vi "Main - Add EtherCAT Master.vi"(8 "error in (no error)":errorcluster, 11 "Node Ptr":u64 format="%.0x") -> (0 "error out":errorcluster)   [LabVIEW 2019, in "SEECD System Explorer.lvlib"]
uses:
  SEECD System Explorer.lvlib
  Shared/Globals/Scan Engine GUIDs.vi
  Shared/Globals/Property Strings.vi
  <vilib>/NI VeriStand/Custom Device API/Custom Device API.lvlib
  Shared/SEECD Shared.lvlib
panel:
  in  "Tag":string
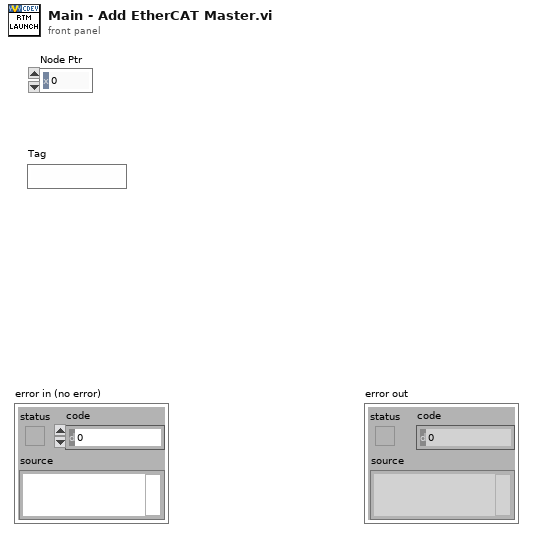
[diagram p1: front panel]
types:
  T1 = typedef "Custom Device API.lvlib/Custom Device Item Ref.ctl" = u64
  T2 = typedef "Custom Device API.lvlib/Custom Device Item Info.ctl" = cluster{"Name":string, "Is Channel":bool, "GUID":string, "Is Waveform":bool}
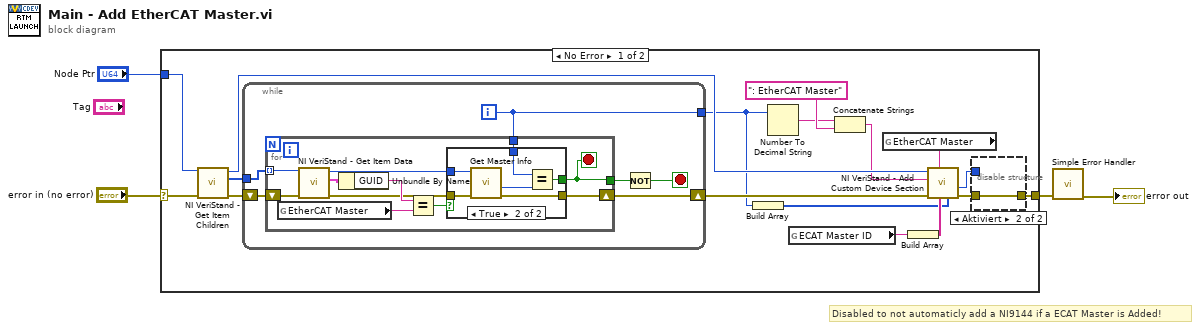
[diagram p0: block diagram]
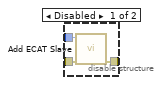
[diagram p2: hidden frame]
diagram:
  # "Disabled to not automaticly add a NI9144 if a ECAT Master is Added!"
  n1 = case shown="No Error" "error in (no error)" {
    selector: "error in (no error)" -> [w21 w50]
    tunnel: "Node Ptr" -> [w20 _]
    tunnel: [w19 w50] -> w2
    frame No Error {
      n2 = call <vilib>:"NI VeriStand - Get Item Children.vi"("error in (no error)"=w21, "Item Ref in"=w20) -> ("error out"=w18:errorcluster, "Child Refs"=w17:T1[], "Item Ref out"=w14:T1)  [unwired: 6 in, 1 out]
      n3 = while {
        shift-right: [w27] -> w15
        shift-left: w18 -> [w31]
        tunnel: w17 -> [w30]
        tunnel: [w26] -> w10
        i -> [w26]
        stop <- w28 stop-if-true
        n4 = for {
          tunnel: w30 -> [w37] mode=indexing
          shift-right: [w40] -> w27
          shift-left: w31 -> [w38]
          tunnel: w26 -> [w42]
          tunnel: [w41] -> w29
          stop <- w41 stop-if-true
          n5 = global read "Scan Engine GUIDs.vi" "EtherCAT Master"() -> (w35:string)
          n6 = call <vilib>:"NI VeriStand - Get Item Data.vi"("error in (no error)"=w38, "Item Ref in"=w37) -> ("error out"=w34:errorcluster, "Item Info"=w39:T2, "Item Ref out"=w33:T1)  [unwired: 6 in, 1 out]
          n7 = Unbundle By Name(w39) -> ("GUID"=w36:string)
          n8 = Equal?(x=w36, y=w35) -> (x = y?=w32:bool)
          n9 = case shown="True" w32 {
            tunnel: w42 -> [_ w49]
            tunnel: [_ w48] -> w41
            tunnel: [w43 w47] -> w40
            tunnel: w34 -> [w43 w45]
            tunnel: w33 -> [_ w44]
            frame False {
            }
            frame True {
              n10 = call "Get Master Info.vi"("error in (no error)"=w45, "Item Ref in"=w44) -> ("error out"=w47:errorcluster, "Master #"=w46:u32)  [unwired: 6 in, 2 out]
              n11 = Equal?(x=w49, y=w46) -> (x = y?=w48:bool)
            }
          }
        }
        n12 = Not(x=w29) -> (.not. x?=w28:bool)
      }
      n13 = Build Array(w10) -> (w11:i32[])
      n14 = Number To Decimal String(number=w10) -> (decimal integer string=w8:string)  [unwired: 1 in]
      n15 = global read "Property Strings.vi" "ECAT Master ID"() -> (w13:string)
      n16 = Concatenate Strings(w8, ": EtherCAT Master" ("string")) -> (w7:string)
      n17 = global read "Scan Engine GUIDs.vi" "EtherCAT Master"() -> (w16:string)
      n18 = Build Array(w13) -> (w12:string[])
      n19 = call <vilib>:"NI VeriStand - Add Custom Device Section.vi"("Property Values"=w11, "Property names"=w12, "GUID (Default Section)"=w16, "error in (no error)"=w15, "Section Name"=w7, "Parent Ref in"=w14) -> ("error out"=w6:errorcluster, "Section Ptr"=w5:T1)  [unwired: 2 in, 2 out]
      n20 = disable-structure shown="Aktiviert" {
        disable-tunnel: [w24 w25] -> w19
        disable-tunnel: w6 -> [w23 w25]
        disable-tunnel: w5 -> [w22 _]
        frame Disabled {
          n21 = call "Add ECAT Slave.vi"("error in (no error)"=w23, "ECAT Master Ref in"=w22) -> ("error out"=w24:errorcluster)  [unwired: 8 in, 1 out]
        }
        frame Enabled {
        }
      }
    }
    frame Error {
    }
  }
  n22 = call <vilib>:"Simple Error Handler.vi"("error in (no error)"=w2) -> ("error out"=→"error out":errorcluster)  [unwired: 4 in, 4 out]
